vi "set crate.vi"(0 "VISA in":refnum<visa-resource-name>, 1 "Location Cluster in":T1, 2 "set crate":i32, 5 "error in":errorcluster) -> (14 "VISA out":refnum<visa-resource-name>, 15 "Location Cluster out":T1, 19 "error out":errorcluster)   [LabVIEW 2018]
uses:
  location cluster.ctl
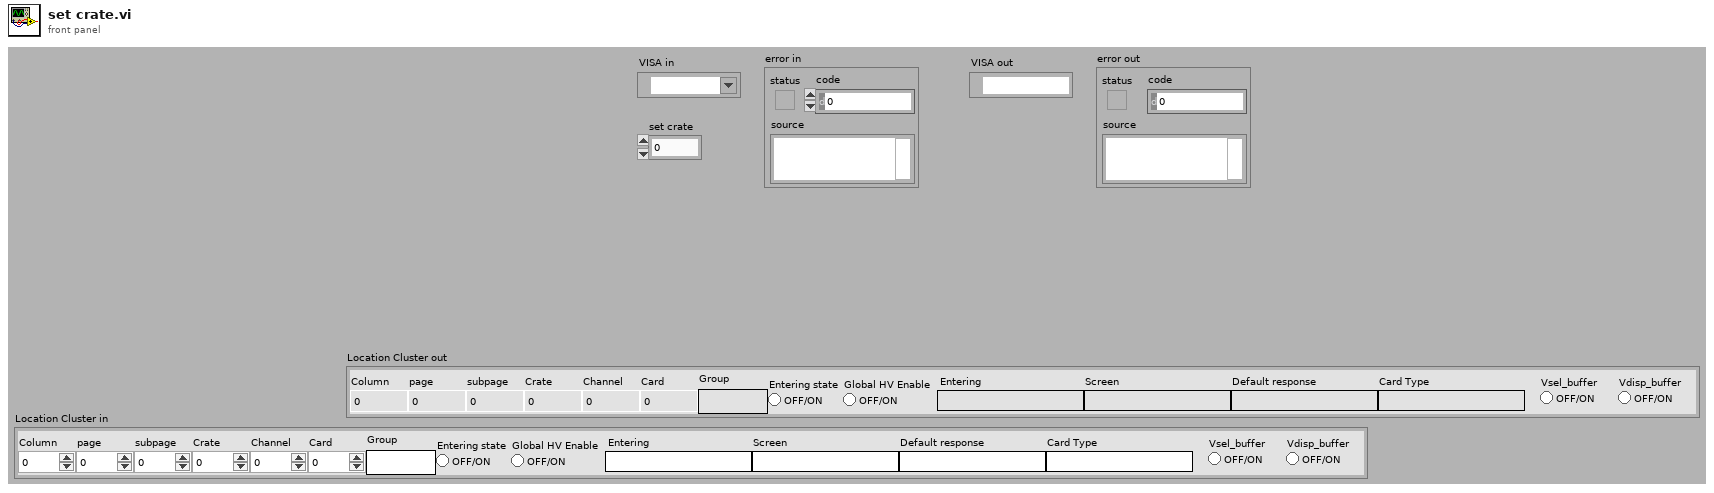
[diagram p1: front panel]
types:
  T1 = typedef "location cluster.ctl" = cluster{"Column":i32, "Card Type":string, "Channel":i32, "Card":i32, "Default response":string, "Entering":string, "Entering state":bool, "subpage":i32, "page":i32, "Crate":i32, "Screen":string, "Group":string, "Global HV Enable":bool, "Vsel_buffer":bool, "Vdisp_buffer":bool}
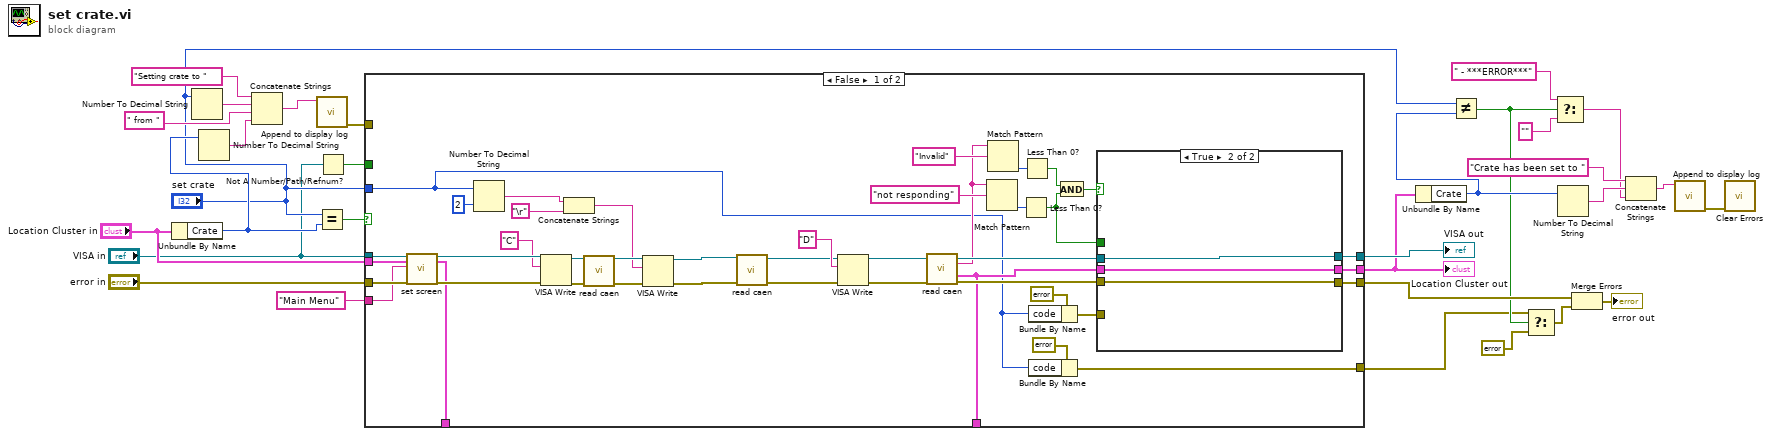
[diagram p0: block diagram]
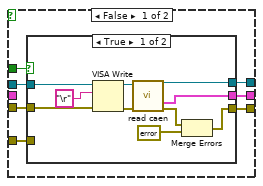
[diagram p2: hidden frame]
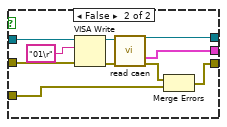
[diagram p3: hidden frame]
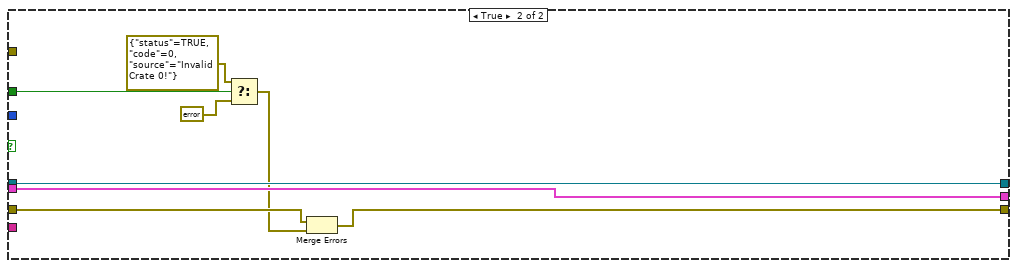
[diagram p4: hidden frame]
diagram:
  n1 = Unbundle By Name("Location Cluster in") -> ("Crate"=w14:i32)
  n2 = Number To Decimal String(number="set crate") -> (decimal integer string=w23:string)  [unwired: 1 in]
  n3 = Number To Decimal String(number=w14) -> (decimal integer string=w15:string)  [unwired: 1 in]
  n4 = Concatenate Strings("Setting crate to " ("string"), w23, " from " ("string"), w15) -> (w22:string)
  n5 = call "Append to display log.vi"("string"=w22) -> ("error out"=w25:errorcluster)  [unwired: 10 in]
  n6 = Equal?(x="set crate", y=w14) -> (x = y?=w27:bool)
  n7 = Not A Number/Path/Refnum?(number/path/refnum="VISA in") -> (NaN/Path/Refnum?=w26:bool)
  n8 = case shown="False" w27 {
    tunnel: "VISA in" -> [w72 w110]
    tunnel: "Location Cluster in" -> [w70 w109]
    tunnel: "error in" -> [w71 w108]
    tunnel: "set crate" -> [w40 _]
    tunnel: [w65 w110] -> w30
    tunnel: [w64 w107] -> w8
    tunnel: [w63 w109] -> w21
    tunnel: [w53 _] -> _
    tunnel: [w52 _] -> _
    tunnel: w26 -> [_ w106]
    tunnel: w25 -> [_ _]
    tunnel: [w39 _] -> w4
    tunnel: "Main Menu" ("set Screen") -> [w36 _]
    frame False {
      n9 = call "set screen.vi"("VISA in"=w72, "Location Cluster in"=w70, "set Screen"=w36, "error in"=w71) -> ("VISA out"=w69:refnum<visa-resource-name>, "Location Cluster out"=w53:T1, "error out"=w54:errorcluster)  [unwired: 13 in]
      n10 = Number To Decimal String(number=w40, width (-)=i16 2) -> (decimal integer string=w43:string)
      n11 = VISA Write(VISA resource name=w69, write buffer="C" ("string"), error in (no error)=w54) -> (VISA resource name out=w45:refnum<visa-resource-name>, error out=w48:errorcluster)  [unwired: 1 out]
      n12 = Concatenate Strings(w43, "\r") -> (w42:string)
      n13 = call "read caen.vi"("VISA in"=w45, "error in"=w48) -> ("VISA out"=w46:refnum<visa-resource-name>, "error out"=w47:errorcluster)  [unwired: 8 in, 4 out]
      n14 = VISA Write(VISA resource name=w46, write buffer=w42, error in (no error)=w47) -> (VISA resource name out=w33:refnum<visa-resource-name>, error out=w34:errorcluster)  [unwired: 1 out]
      n15 = call "read caen.vi"("VISA in"=w33, "error in"=w34) -> ("VISA out"=w31:refnum<visa-resource-name>, "error out"=w32:errorcluster)  [unwired: 8 in, 4 out]
      n16 = VISA Write(VISA resource name=w31, write buffer="D" ("string"), error in (no error)=w32) -> (VISA resource name out=w38:refnum<visa-resource-name>, error out=w35:errorcluster)  [unwired: 1 out]
      n17 = call "read caen.vi"("VISA in"=w38, "error in"=w35) -> ("VISA out"=w66:refnum<visa-resource-name>, "Read string"=w56:string, "Location Cluster"=w52:T1, "error out"=w67:errorcluster)  [unwired: 8 in, 2 out]
      n18 = Match Pattern(string=w56, regular expression="not responding" ("search string")) -> (offset past match=w60:i32)  [unwired: 1 in, 3 out]
      n19 = Match Pattern(string=w56, regular expression="Invalid" ("search string")) -> (offset past match=w61:i32)  [unwired: 1 in, 3 out]
      n20 = Less Than 0?(x=w60) -> (x < 0?=w55:bool)
      n21 = Less Than 0?(x=w61) -> (x < 0?=w58:bool)
      n22 = Bundle By Name(cluster=errorcluster {"status"=TRUE, "code"=0, "source"="Crate not responding!"} ("error in"), "code"=w40) -> (w50:errorcluster)
      n23 = Bundle By Name(cluster=errorcluster {"status"=TRUE, "code"=0, "source"="Failed to set crate"} ("error in"), "code"=w40) -> (w39:errorcluster)
      n24 = And(x=w58, y=w55) -> (x .and. y?=w57:bool)
      n25 = case shown="True" w57 {
        tunnel: w67 -> [w79 w101]
        tunnel: w66 -> [w78 w102]
        tunnel: [w77 w102] -> w65
        tunnel: [w75 w101] -> w64
        tunnel: [w76 w100] -> w63
        tunnel: w52 -> [_ w100]
        tunnel: w55 -> [w74 _]
        tunnel: w50 -> [w73 _]
        frame False {
          n26 = case shown="True" w74 {
            tunnel: w79 -> [w89 w99]
            tunnel: w78 -> [w88 w98]
            tunnel: [w84 w94] -> w77
            tunnel: [w83 w93] -> w76
            tunnel: [w80 w91] -> w75
            tunnel: w73 -> [_ w90]
            frame True {
              n27 = VISA Write(VISA resource name=w88, write buffer="\r" ("search string"), error in (no error)=w89) -> (VISA resource name out=w85:refnum<visa-resource-name>, error out=w86:errorcluster)  [unwired: 1 out]
              n28 = call "read caen.vi"("VISA in"=w85, "error in"=w86) -> ("VISA out"=w84:refnum<visa-resource-name>, "Location Cluster"=w83:T1, "error out"=w81:errorcluster)  [unwired: 8 in, 3 out]
              n29 = Merge Errors(w81, errorcluster {"status"=TRUE, "code"=0, "source"="Invalid Crate!"} ("error in")) -> (w80:errorcluster)
            }
            frame False {
              n30 = VISA Write(VISA resource name=w98, write buffer="01\r" ("search string"), error in (no error)=w99) -> (VISA resource name out=w95:refnum<visa-resource-name>, error out=w96:errorcluster)  [unwired: 1 out]
              n31 = call "read caen.vi"("VISA in"=w95, "error in"=w96) -> ("VISA out"=w94:refnum<visa-resource-name>, "Location Cluster"=w93:T1, "error out"=w92:errorcluster)  [unwired: 8 in, 3 out]
              n32 = Merge Errors(w92, w90) -> (w91:errorcluster)
            }
          }
        }
        frame True {
        }
      }
    }
    frame True {
      n33 = Select(t=errorcluster {"status"=TRUE, "code"=0, "source"="Invalid Crate 0!"} ("error in"), s=w106, f=errorcluster {"status"=FALSE, "code"=0, "source"=""}) -> (s? t:f=w103:errorcluster)
      n34 = Merge Errors(w108, w103) -> (w107:errorcluster)
    }
  }
  "Location Cluster out" <- w21
  "VISA out" <- w30
  n35 = Unbundle By Name(w21) -> ("Crate"=w11:i32)
  n36 = Not Equal?(x="set crate", y=w11) -> (x != y?=w5:bool)
  n37 = Select(t=w4, s=w5, f=errorcluster {"status"=FALSE, "code"=0, "source"=""} ("t")) -> (s? t:f=w6:errorcluster)
  n38 = Select(t=" - ***ERROR***" ("string"), s=w5, f="" ("string")) -> (s? t:f=w9:string)
  n39 = Number To Decimal String(number=w11) -> (decimal integer string=w20:string)  [unwired: 1 in]
  n40 = Merge Errors(w8, w6) -> (→"error out":errorcluster)
  n41 = Concatenate Strings("Crate has been set to " ("string"), w20, w9) -> (w18:string)
  n42 = call "Append to display log.vi"("string"=w18) -> ("error out"=w17:errorcluster)  [unwired: 10 in]
  n43 = call <vilib>:"Clear Errors.vi"("error in (no error)"=w17) -> ()  [unwired: 5 in, 2 out]
